vi "initialize.vi"(0 "MyApp":refnum<class "MyApp.lvclass">, 3 "initializationData":variant, 5 "error in (no error)":errorcluster, 7 "binaryString":string, 8 "I8 Array":i8[](array[numeric]), 9 "prependSize? (T)":bool, 11 "byteOrder (0:big-endian, network order)":T1(ring)) -> (14 "dup MyApp":refnum<class "MyApp.lvclass">, 17 "found?":bool, 19 "error out":errorcluster)   [LabVIEW 2012, in "MyApp.lvlib" / "MyApp.lvclass"]
doc: "This is a dynamic dispatch VI to be implemented by child classes to initialize their attributes.\n\n<B>Recommendation:</B> Use Variant for initialization data."
uses:
  MyApp.lvclass
  MyAppConfig.lvclass
  HGF_LVC/HGF_ApplicationBaseClasses/HGF_Application/HGF_Application.lvclass
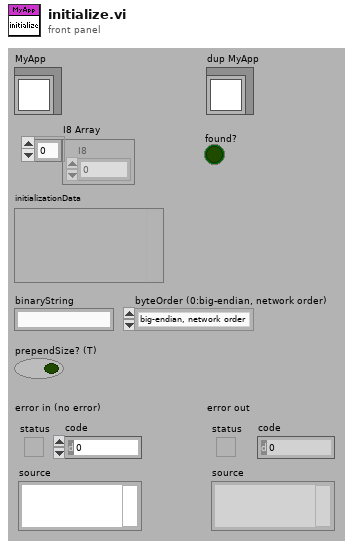
[diagram p1: front panel]
types:
  T1 = enum16{"big-endian, network order", "native, host order", "little-endian"}
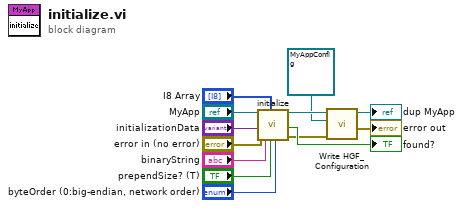
[diagram p0: block diagram]
diagram:
  n1 = call-parent "initialize.vi"("HGF_Factory"="MyApp", "initializationData"="initializationData", "error in (no error)"="error in (no error)", "binaryString"="binaryString", "I8 Array"="I8 Array", "prependSize? (T)"="prependSize? (T)", "byteOrder (0:big-endian, network order)"="byteOrder (0:big-endian, network order)") -> ("dup HGF_Factory"=w5:refnum<class "MyApp.lvclass">, "found?"=→"found?":bool, "error out"=w3:errorcluster)  [unwired: 10 in]
  n2 = call "Write HGF_Configuration.vi"("error in (no error)"=w3, "HGF_Configuration"=refnum<class "MyAppConfig.lvclass"> refnum ("MyAppConfig.lvclass"), "HGF_Application in"=w5) -> ("error out"=→"error out":errorcluster, "HGF_Application out"=→"dup MyApp":refnum<class "MyApp.lvclass">)  [unwired: 7 in]
